vi "Set Variable Engine.vi"(8 "error in (no error)":errorcluster, 10 "Variable Engine":refnum<class "Variable Engine.lvclass">, 11 "App Properties in":refnum<class "App Properties.lvclass">) -> (0 "error out":errorcluster, 3 "App Properties out":refnum<class "App Properties.lvclass">)   [LabVIEW 2017, in "Application.lvlib" / "App Properties.lvclass"]
uses:
  App Properties.lvclass
  <vilib>/TSS/ACRObat Test Framework/Classes/Variable Engine/Class/Variable Engine.lvclass
  App Properties.lvclass/App Properties.ctl
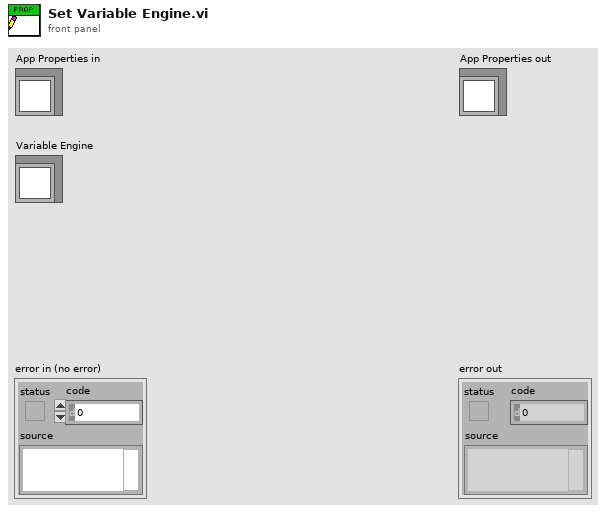
[diagram p1: front panel]
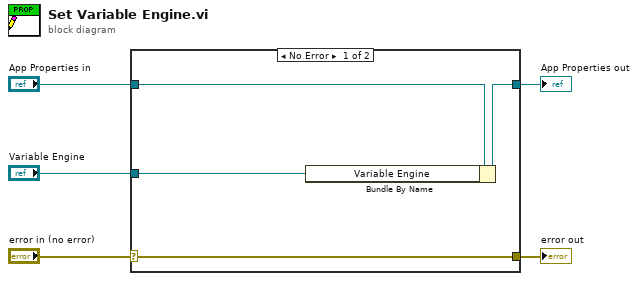
[diagram p0: block diagram]
diagram:
  n1 = case shown="No Error" "error in (no error)" {
    selector: "error in (no error)" -> [w9 w10]
    tunnel: [w9 w10] -> w4
    tunnel: [w7 w11] -> w2
    tunnel: "App Properties in" -> [w8 w11]
    tunnel: "Variable Engine" -> [w6 _]
    frame No Error {
      n2 = Bundle By Name(cluster=w8, "Variable Engine"=w6) -> (w7:refnum<class "App Properties.lvclass">)
    }
    frame Error {
    }
  }
  "error out" <- w4
  "App Properties out" <- w2
